vi "ma_format To Audio Data Format.vi"(11 "ma_format":u16) -> (3 "Format":T1)   [LabVIEW 2020, in "G-Audio.lvlib"]
uses:
  Controls/Audio Device Format.ctl
  G-Audio.lvlib
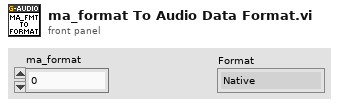
[diagram p1: front panel]
types:
  T1 = typedef "G-Audio.lvlib/Audio Device Format.ctl" = enum16{"Native", "U8", "I16", "I32", "SGL"}
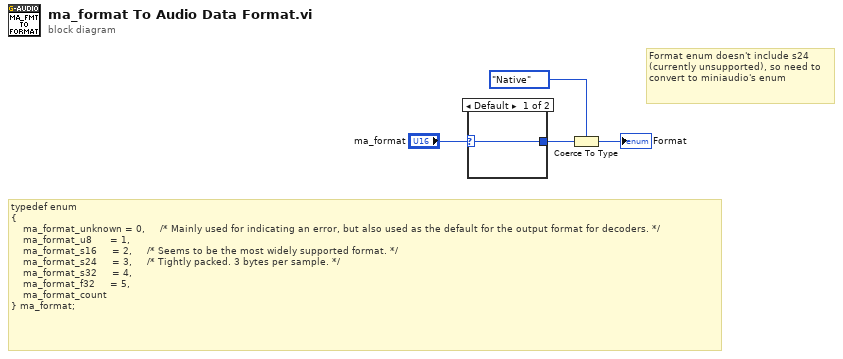
[diagram p0: block diagram]
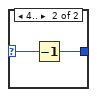
[diagram p2: hidden frame]
diagram:
  # "Format enum doesn't include s24 (currently unsupported), so need to convert to miniaudio's enum"
  # "typedef enum\n{\n    ma_format_unknown = 0,     /* Mainly used for indicating an error, but also used as the default for the output format for decoders. */\n    ma_format_u8      = 1,\n    ma_format_s16     = 2,     /* Seems to be the most widely supported format. */\n    ma_format_s24     = 3,     /* Tightly packed. 3 bytes per sample. */\n    ma_format_s32     = 4,\n    ma_format_f32     = 5,\n    ma_format_count\n} ma_format;"
  n1 = case shown="Default" "ma_format" {
    selector: "ma_format" -> [w5 w7]
    tunnel: [w5 w6] -> w3
    frame Default {
    }
    frame 4.. {
      n2 = Decrement(x=w7) -> (x-1=w6:u16)
    }
  }
  n3 = Coerce To Type(0:w3, 1:Audio_Device_Format."Native" ("Format")) -> (2:→"Format":T1)
